vi "Set File Permissions.vi"(6 "Permissions":T1 items=["Read Only"=292, "Read/Write"=438], 8 "error in":errorcluster, 11 "File Path":path) -> (0 "error out":errorcluster, 3 "File Path.DUP":path)   [LabVIEW 2024]
uses:
  File Permissions Selector.ctl
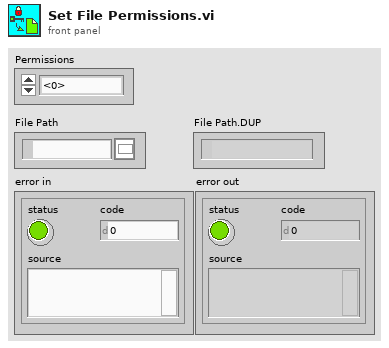
[diagram p1: front panel]
types:
  T1 = typedef "File Permissions Selector.ctl" = i16
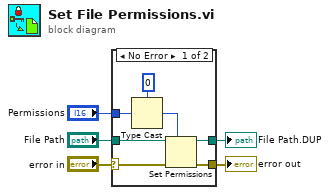
[diagram p0: block diagram]
diagram:
  n1 = case shown="No Error" "error in" {
    selector: "error in" -> [w6 w13]
    tunnel: [w12 w13] -> w5
    tunnel: "Permissions" -> [w11 _]
    tunnel: "File Path" -> [w10 _]
    tunnel: [w7 _] -> w2
    frame No Error {
      n2 = Type Cast(type=i16 0, x=w11) -> (*(type *) &x=w9:i16)
      n3 = Set Permissions(7:w9, 8:w6, 11:w10) -> (0:w12:errorcluster, 3:w7:path)  [unwired: 2 in]
    }
    frame Error {
    }
  }
  "error out" <- w5
  "File Path.DUP" <- w2
